vi "CRYAna Single Side Spectrum.vi"(10 "FFT Size":i32=2, 11 "FFT":cdb[](array[numeric]) format="%#.6g") -> (2 "Spectrum Size":i32=2, 3 "Single FFT":cdb[](array[numeric]) format="%#_7g")   [LabVIEW 2013]
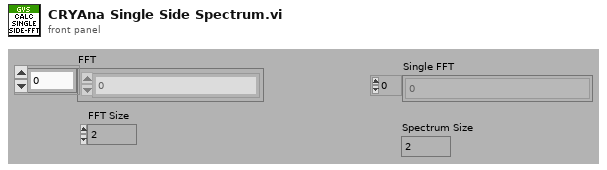
[diagram p1: front panel]
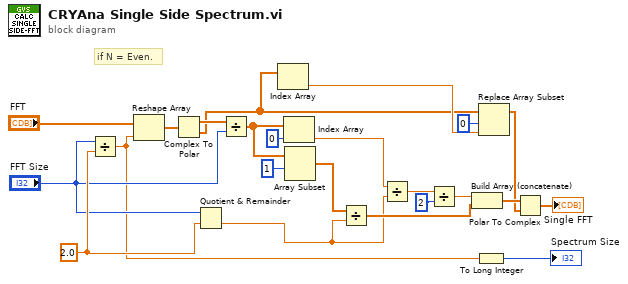
[diagram p0: block diagram]
diagram:
  w10 = 2.0 ("x")
  # "if N = Even."
  n1 = Divide(x="FFT Size", y=w10) -> (x/y=w5:dbl)
  n2 = Reshape Array("FFT", w5) -> (w4:cdb[])
  n3 = Complex To Polar(r * e^(i*theta)=w4) -> (r=w16:dbl[], theta=w2:dbl[])
  n4 = Quotient & Remainder(x="FFT Size", y=w10) -> (floor(x/y)=w11:dbl)  [unwired: 1 out]
  n5 = Divide(x=w16, y="FFT Size") -> (x/y=w19:dbl[])
  n6 = Index Array(array=w2) -> (element=w3:dbl)  [unwired: 1 in]
  n7 = Index Array(array=w19, index=0) -> (element=w7:dbl)
  n8 = Array Subset(array=w19, index=1) -> (w18:dbl[])  [unwired: 1 in]
  n9 = Divide(x=w18, y=w11) -> (x/y=w21:dbl[])
  n10 = Divide(x=w7, y=w11) -> (x/y=w8:dbl)
  n11 = Divide(x=w8, y=2 ("x")) -> (x/y=w6:dbl)
  n12 = Build Array (concatenate)(w6, w21) -> (w17:dbl[])
  n13 = To Long Integer(number=w5) -> (32bit integer=→"Spectrum Size":i32)
  n14 = Replace Array Subset(array=w2, new element=w3, index=0) -> (w13:dbl[])
  n15 = Polar To Complex(1:w13, 2:w17) -> (0:→"Single FFT":cdb[])
